vi "bac.vi"() -> ()   [LabVIEW 2019]
uses:
  <vilib>/Rock Robotics/WPI/ThirdParty/Phoenix-LabVIEW/Motor Controller/Controls/CTRE_Phoenix_MotorControl_ControlMode.ctl
  <vilib>/Rock Robotics/WPI/ThirdParty/Phoenix-LabVIEW/Motor Controller/Get/CTRE_Phoenix_MotorController_GetQuadratureData.vi
  <vilib>/Rock Robotics/Network Tables/NT Read Boolean.vi
  <vilib>/Rock Robotics/Network Tables/NT Read Number.vi
  Robot Global Data.vi
  <vilib>/Rock Robotics/Network Tables/NT Write Boolean.vi
  <vilib>/Rock Robotics/Network Tables/NT Write Number.vi
panel:
  out "Quadrature Position":i32
  out "Switch Pressed 3":bool
  out "Switch Pressed 2":bool
  out "Switch Pressed":bool
  in  "State":i8
  in  "Motor Speed":dbl=1.0
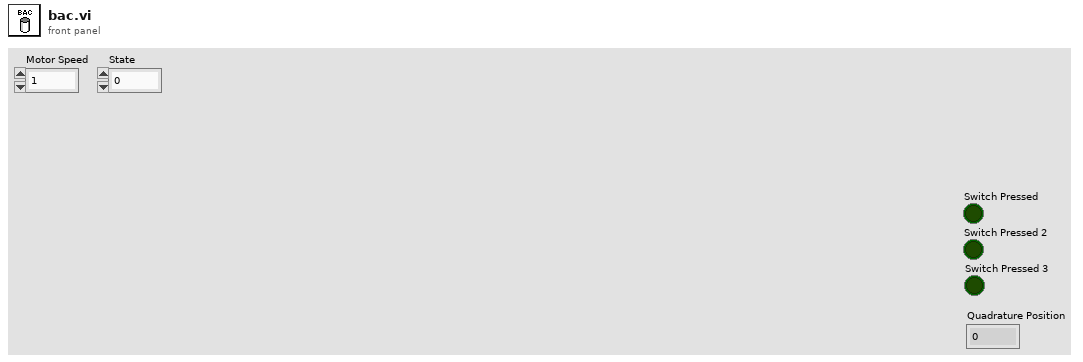
[diagram p1: front panel]
types:
  T1 = typedef "CTRE_Phoenix_MotorControl_ControlMode.ctl" = u16
  T2 = typedef "WPI_SwitchDevRef.ctl" = cluster{"DevStatus":errorcluster, "DIO Channel":T3, "CntIndex":T4, "Normally Closed":bool}
  T3 = typedef "FPGA_DIOChannel.ctl" = enum8{"DIO 0", "DIO 1", "DIO 2", "DIO 3", "DIO 4", "DIO 5", "DIO 6", "DIO 7", "DIO 8", "DIO 9", "DIO MXP 0", "DIO MXP 1", "DIO MXP 2", "DIO MXP 3", "DIO MXP 4", "DIO MXP 5", "DIO MXP 6", "DIO MXP 7", "DIO MXP 8", "DIO MXP 9", "DIO MXP 10", "DIO MXP 11", "DIO MXP 12", "DIO MXP 13", "DIO MXP 14", "DIO MXP 15", "SPI Port CS1", "SPI Port CS2", "SPI Port CS3", "SPI Port MISO", "SPI Port MOSI", "Invalid"}
  T4 = typedef "FPGA_CounterCtrSystemIndex.ctl" = enum8{"Ctr 0", "Ctr 1", "Ctr 2", "Ctr 3", "Ctr 4", "Ctr 5", "Ctr 6", "Ctr 7", "Invalid"}
  T5 = typedef "WPI_MotorControlDeviceRef.ctl" = cluster{"DeviceStatus":errorcluster, "Type":T6, "PWM":cluster{"PWM Channel":T7, "DeadBand":T8}, "CAN":cluster{"Device Number":u8, "SetOutput VI Ref":variant, "GetOutput VI Ref":variant, "Enable VI Ref":variant, "Disable VI Ref":variant, "Data":variant}, "Invert":bool, "DIO PWM":cluster{"PWM \"Enable\" Channel":T7, "DIOChannel":T3, "PWM Rate":dbl}}
  T6 = typedef "WPI_MotorControlType.ctl" = enum16{"PWM", "CAN", "DIO PWM"}
  T7 = typedef "FPGA_DIOPWMChannel.ctl" = enum8{"PWM 0", "PWM 1", "PWM 2", "PWM 3", "PWM 4", "PWM 5", "PWM 6", "PWM 7", "PWM 8", "PWM 9", "PWM MXP 0", "PWM MXP 1", "PWM MXP 2", "PWM MXP 3", "PWM MXP 4", "PWM MXP 5", "PWM MXP 6", "PWM MXP 7", "PWM MXP 8", "PWM MXP 9", "Invalid"}
  T8 = typedef "WPI_PWMDeadband.ctl" = cluster{"Name":string, "maxPositivePwm":i32, "minPositivePwm":i32, "centerPwm":i32, "maxNegativePwm":i32, "minNegativePwm":i32, "angularRange":u16}
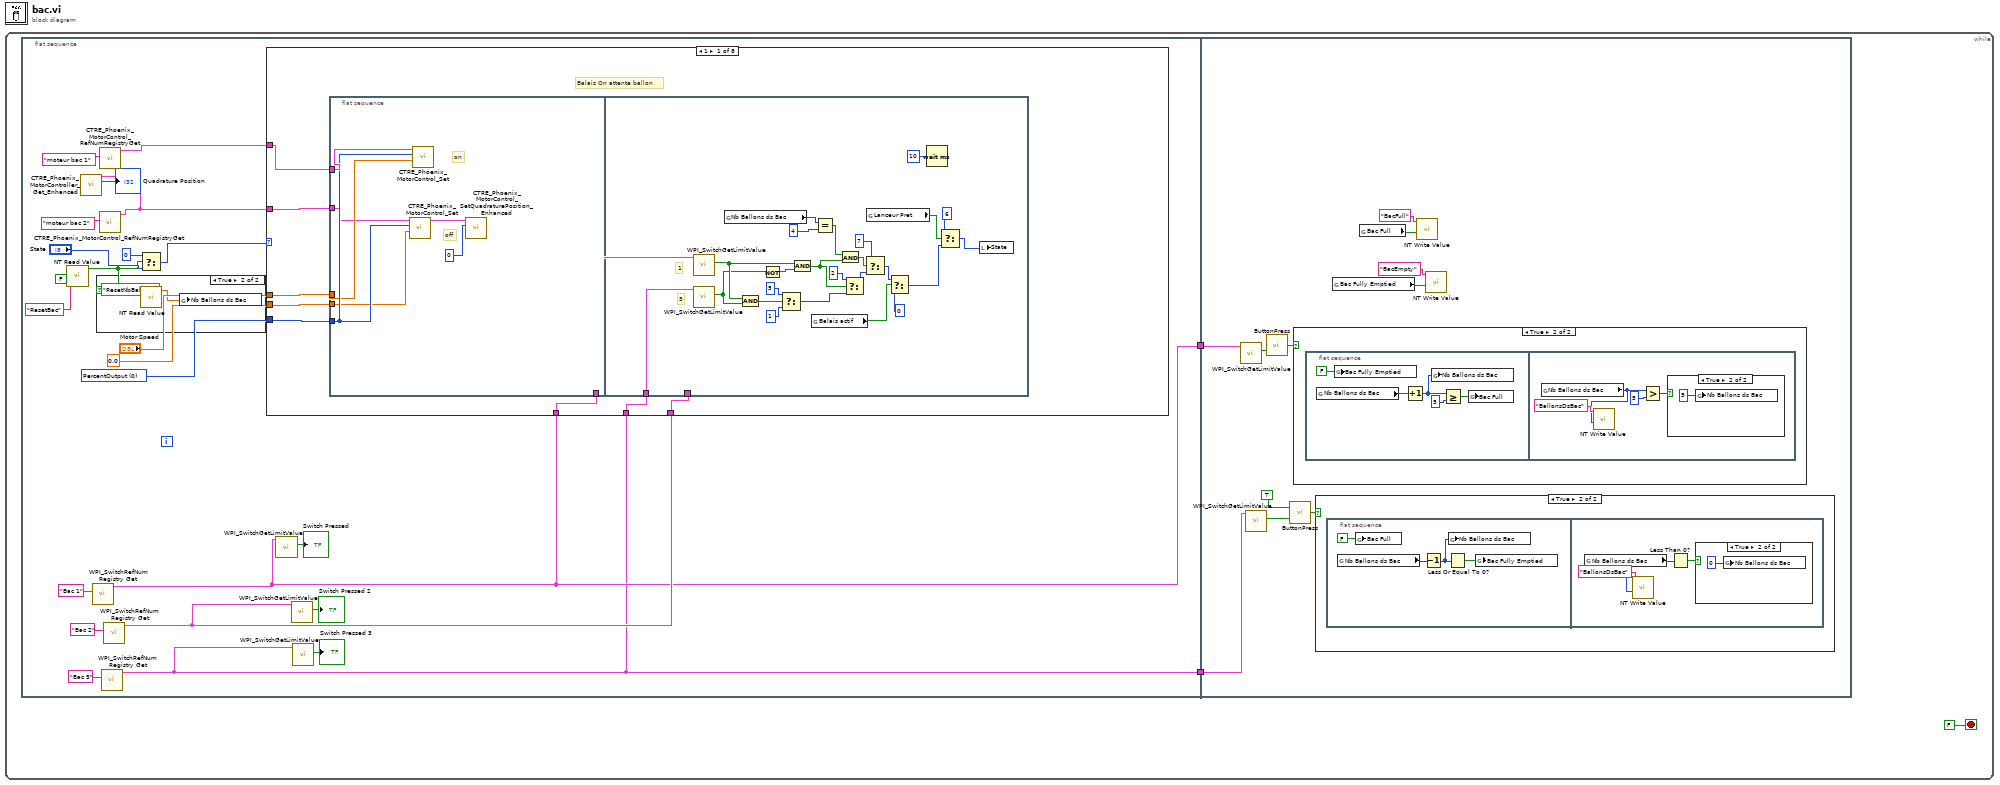
[diagram p0: block diagram]
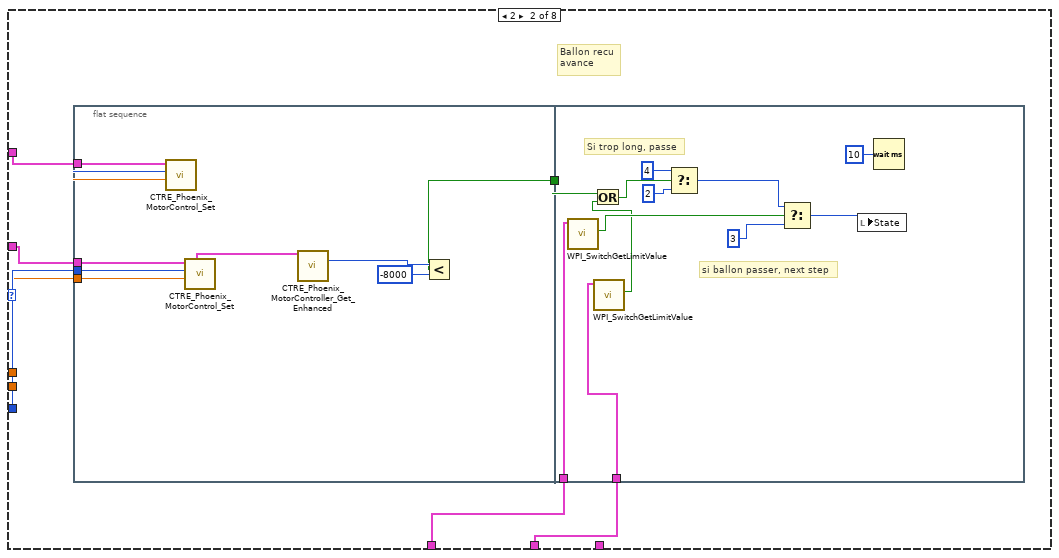
[diagram p3: hidden frame]
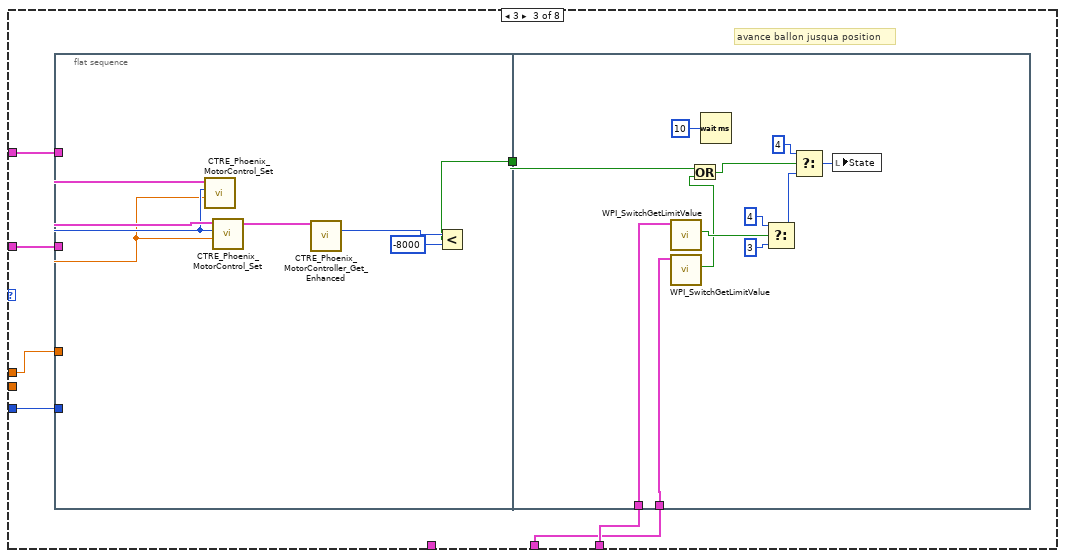
[diagram p4: hidden frame]
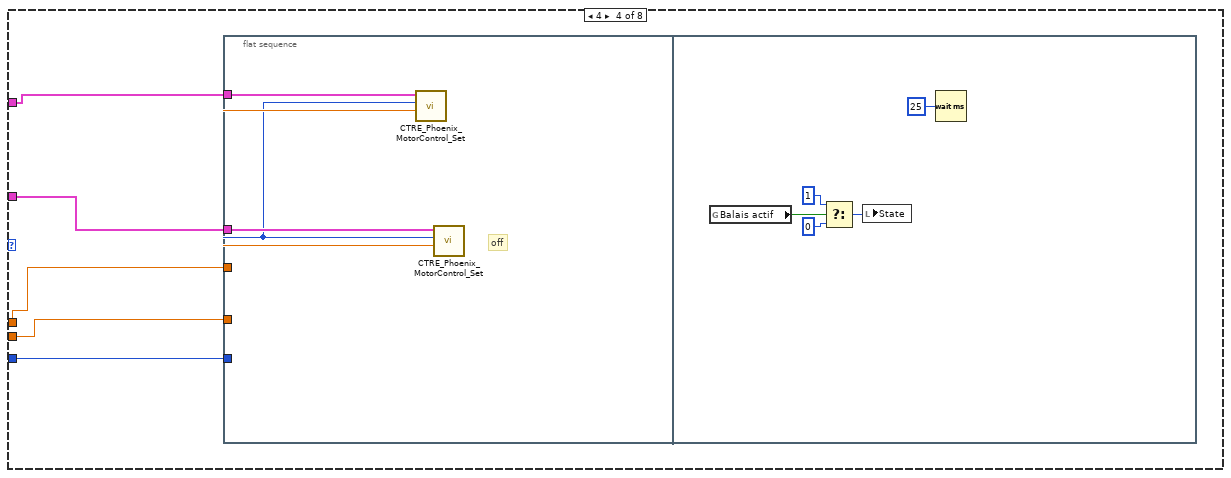
[diagram p5: hidden frame]
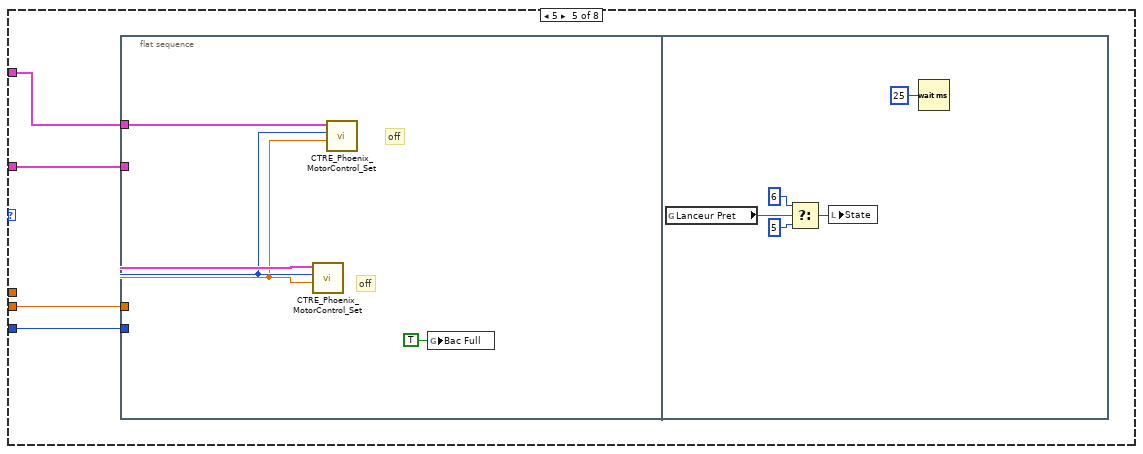
[diagram p6: hidden frame]
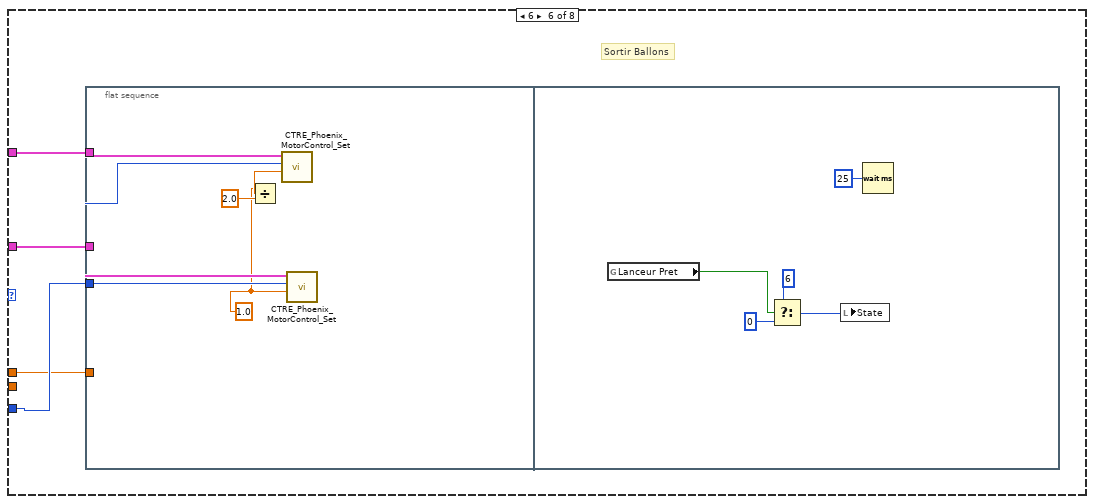
[diagram p7: hidden frame]
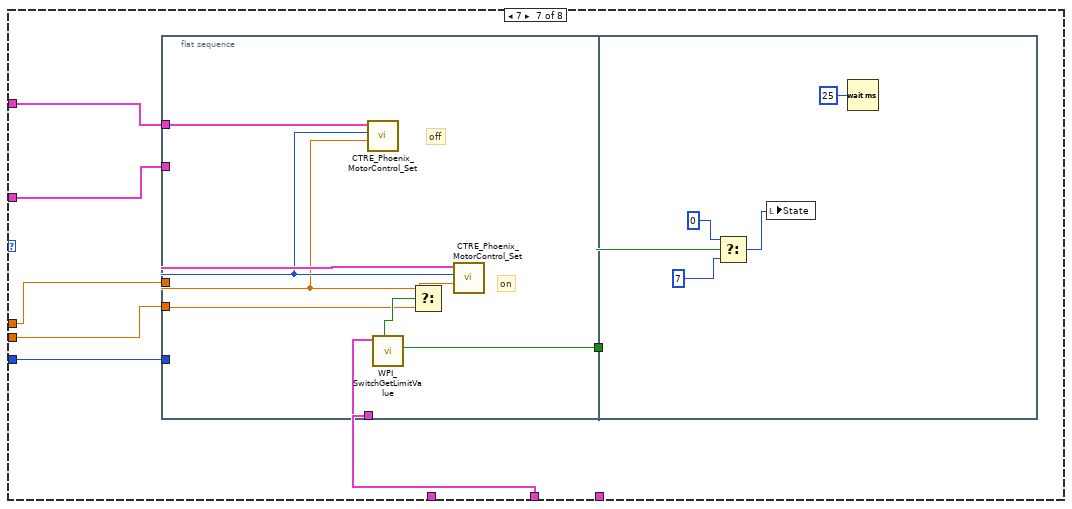
[diagram p8: hidden frame]
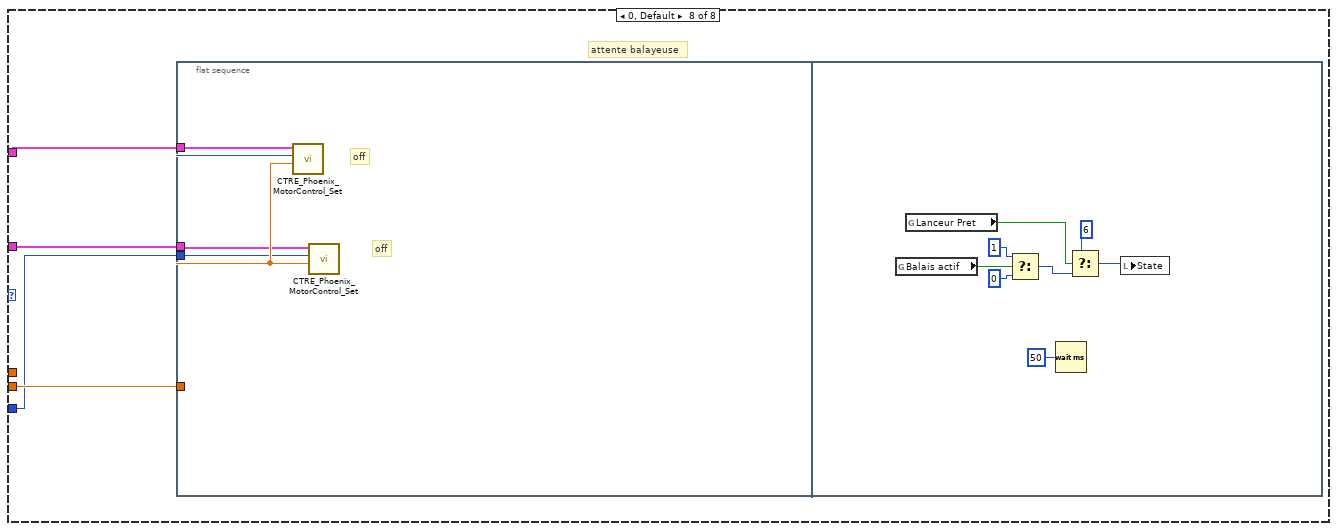
[diagram p9: hidden frame]
diagram:
  n1 = while {
    stop <- FALSE stop-if-true
    n2 = flat-sequence {
      tunnel: [w14] -> w2
      tunnel: [w11] -> w1
      tunnel: w2 -> [w208]
      tunnel: w1 -> [w207]
      frame #0 {
        w23 = T1 0 items=["PercentOutput"=0, "Position"=1, "Velocity"=2, "Current"=3, "Follower"=5, "MotionProfile"=6, "MotionMagic"=7, "MotionProfileArc"=10, "Disabled"=15] ("Control Mode")
        n3 = call-poly <vilib>:"NT Read Value.vi"("Default Value"=FALSE, "Name"="ResetBac") -> ("Boolean"=w4:bool)  [unwired: 8 in, 1 out]
        n4 = call <vilib>:"WPI_SwitchRefNum Registry Get.vi"("refnum name"="Bac 1") -> ("SwitchDevRef"=w14:T2)  [unwired: 9 in, 1 out]
        n5 = case shown="True" w4 {
          frame False {
          }
          frame True {
            n6 = call-poly <vilib>:"NT Read Value.vi"("Name"="ResetNbBallon") -> ("Numeric"=w27:dbl)  [unwired: 9 in, 1 out]
            n7 = global write "Robot Global Data.vi" "Nb Ballons ds Bac"(w27) -> ()
          }
        }
        n8 = call <vilib>:"CTRE_Phoenix_MotorControl_RefNumRegistryGet.vi"("refnum name"="moteur bac 2") -> ("PhoenixMotorControlDevRef"=w17:T5)  [unwired: 9 in, 1 out]
        n9 = call-poly <vilib>:"CTRE_Phoenix_MotorController_Get_Enhanced.vi"("PhoenixMotorControlDevRef"=w17) -> ("Quadrature Position"=→"Quadrature Position":i32)  [unwired: 11 in, 3 out]
        n10 = call <vilib>:"CTRE_Phoenix_MotorControl_RefNumRegistryGet.vi"("refnum name"="moteur bac 1") -> ("PhoenixMotorControlDevRef"=w25:T5)  [unwired: 9 in, 1 out]
        n11 = call <vilib>:"WPI_SwitchRefNum Registry Get.vi"("refnum name"="Bac 5") -> ("SwitchDevRef"=w11:T2)  [unwired: 9 in, 1 out]
        n12 = call <vilib>:"WPI_SwitchRefNum Registry Get.vi"("refnum name"="Bac 2") -> ("SwitchDevRef"=w16:T2)  [unwired: 9 in, 1 out]
        n13 = Select(t=i8 0, s=w4, f="State") -> (s? t:f=w5:i8)
        n14 = case shown="1" w5 {
          tunnel: w25 -> [w36 w75 w102 w126 w141 w155 w173 w190]
          tunnel: w23 -> [w35 w73 w100 w125 w139 w153 w169 w188]
          tunnel: 0.0 -> [w34 _ _ w124 w138 _ w171 w189]
          tunnel: "Motor Speed" -> [w33 w72 w99 w123 _ w152 w170 _]
          tunnel: w11 -> [w32 w69 w96 _ _ _ w168 _]
          tunnel: w17 -> [w30 w74 w101 w127 w140 w154 w172 w187]
          tunnel: w14 -> [w31 w71 _ _ _ _ _ _]
          tunnel: w16 -> [w29 _ w98 _ _ _ _ _]
          frame 1 {
            # "Balais On attente ballon"
            n15 = flat-sequence {
              tunnel: w36 -> [w43]
              tunnel: w35 -> [w42]
              tunnel: w34 -> [w41]
              tunnel: w33 -> [w40]
              tunnel: w30 -> [w39]
              tunnel: w32 -> [w64]
              tunnel: w31 -> [w63]
              tunnel: w29 -> [_]
              frame #0 {
                # "off"
                # "on"
                n16 = call <vilib>:"CTRE_Phoenix_MotorControl_Set.vi"("Output"=w41, "Control Mode"=w42, "PhoenixMotorControlDevRef"=w39) -> ("PhoenixMotorControlDevRef"=w38:T5)  [unwired: 7 in, 1 out]
                n17 = call <vilib>:"CTRE_Phoenix_MotorControl_Set.vi"("Output"=w40, "Control Mode"=w42, "PhoenixMotorControlDevRef"=w43) -> ()  [unwired: 7 in, 2 out]
                n18 = call <vilib>:"CTRE_Phoenix_MotorControl_SetQuadraturePosition_Enhanced.vi"("New Position"=0, "PhoenixMotorControlDevRef"=w38) -> ()  [unwired: 8 in, 2 out]
              }
              frame #1 {
                # "5"
                # "1"
                n19 = call <vilib>:"WPI_SwitchGetLimitValue.vi"("SwitchDevRef"=w63) -> ("Switch Pressed"=w62:bool)  [unwired: 8 in, 2 out]
                n20 = call <vilib>:"WPI_SwitchGetLimitValue.vi"("SwitchDevRef"=w64) -> ("Switch Pressed"=w61:bool)  [unwired: 8 in, 2 out]
                n21 = global read "Robot Global Data.vi" "Nb Ballons ds Bac"() -> (w51:u8)
                n22 = Compound Arithmetic op=AND(w62, w61) -> (w60:bool)
                n23 = Not(x=w61) -> (.not. x?=w65:bool)
                n24 = Select(t=i8 5, s=w60, f=i8 1) -> (s? t:f=w59:i8)
                n25 = And(x=w62, y=w65) -> (x .and. y?=w47:bool)
                n26 = global read "Robot Global Data.vi" "Balais actif"() -> (w54:bool)
                n27 = Equal?(x=w51, y=u8 4) -> (x = y?=w46:bool)
                n28 = And(x=w46, y=w47) -> (x .and. y?=w48:bool)
                n29 = Select(t=i8 2, s=w47, f=w59) -> (s? t:f=w49:i8)
                n30 = Select(t=i8 7, s=w48, f=w49) -> (s? t:f=w44:i8)
                n31 = global read "Robot Global Data.vi" "Lanceur Pret"() -> (w57:bool)
                n32 = Select(t=w44, s=w54, f=i8 0) -> (s? t:f=w53:i8)
                n33 = Wait (ms)(milliseconds to wait=u32 10) -> ()  [unwired: 1 out]
                n34 = Select(t=i8 6, s=w57, f=w53) -> (s? t:f=w55:i8)
                n35 = local write "State"(w55) -> ()
              }
            }
          }
          frame 2 {
            # "Ballon recu\navance"
            n36 = flat-sequence {
              tunnel: w75 -> [w83]
              tunnel: w74 -> [w82]
              tunnel: w73 -> [w81]
              tunnel: w72 -> [w80]
              tunnel: [w76] -> w70
              tunnel: w71 -> [w95]
              tunnel: w70 -> [w87]
              tunnel: w69 -> [w85]
              frame #0 {
                n37 = call <vilib>:"CTRE_Phoenix_MotorControl_Set.vi"("Output"=w80, "Control Mode"=w81, "PhoenixMotorControlDevRef"=w83) -> ()  [unwired: 7 in, 2 out]
                n38 = call <vilib>:"CTRE_Phoenix_MotorControl_Set.vi"("Output"=w80, "Control Mode"=w81, "PhoenixMotorControlDevRef"=w82) -> ("PhoenixMotorControlDevRef"=w77:T5)  [unwired: 7 in, 1 out]
                n39 = call-poly <vilib>:"CTRE_Phoenix_MotorController_Get_Enhanced.vi"("PhoenixMotorControlDevRef"=w77) -> ("Quadrature Position"=w79:i32)  [unwired: 11 in, 3 out]
                n40 = Less?(x=w79, y=-8000) -> (x < y?=w76:bool)
              }
              frame #1 {
                # "si ballon passer, next step"
                # "Si trop long, passe"
                n41 = call <vilib>:"WPI_SwitchGetLimitValue.vi"("SwitchDevRef"=w95) -> ("Switch Pressed"=w88:bool)  [unwired: 8 in, 2 out]
                n42 = call <vilib>:"WPI_SwitchGetLimitValue.vi"("SwitchDevRef"=w85) -> ("Switch Pressed"=w84:bool)  [unwired: 8 in, 2 out]
                n43 = Or(x=w87, y=w84) -> (x .or. y?=w86:bool)
                n44 = Select(t=i8 4, s=w86, f=i8 2) -> (s? t:f=w89:i8)
                n45 = Select(t=w89, s=w88, f=i8 3 ("t")) -> (s? t:f=w92:i8)
                n46 = local write "State"(w92) -> ()
                n47 = Wait (ms)(milliseconds to wait=u32 10) -> ()  [unwired: 1 out]
              }
            }
          }
          frame 3 {
            # "avance ballon jusqua position"
            n48 = flat-sequence {
              tunnel: w102 -> [w110]
              tunnel: w101 -> [w109]
              tunnel: w100 -> [w108]
              tunnel: w99 -> [w107]
              tunnel: [w103] -> w97
              tunnel: w98 -> [w122]
              tunnel: w97 -> [w113]
              tunnel: w96 -> [w115]
              frame #0 {
                n49 = call <vilib>:"CTRE_Phoenix_MotorControl_Set.vi"("Output"=w107, "Control Mode"=w108, "PhoenixMotorControlDevRef"=w110) -> ()  [unwired: 7 in, 2 out]
                n50 = call <vilib>:"CTRE_Phoenix_MotorControl_Set.vi"("Output"=w107, "Control Mode"=w108, "PhoenixMotorControlDevRef"=w109) -> ("PhoenixMotorControlDevRef"=w104:T5)  [unwired: 7 in, 1 out]
                n51 = call-poly <vilib>:"CTRE_Phoenix_MotorController_Get_Enhanced.vi"("PhoenixMotorControlDevRef"=w104) -> ("Quadrature Position"=w106:i32)  [unwired: 11 in, 3 out]
                n52 = Less?(x=w106, y=-8000) -> (x < y?=w103:bool)
              }
              frame #1 {
                n53 = call <vilib>:"WPI_SwitchGetLimitValue.vi"("SwitchDevRef"=w122) -> ("Switch Pressed"=w114:bool)  [unwired: 8 in, 2 out]
                n54 = call <vilib>:"WPI_SwitchGetLimitValue.vi"("SwitchDevRef"=w115) -> ("Switch Pressed"=w111:bool)  [unwired: 8 in, 2 out]
                n55 = Or(x=w113, y=w111) -> (x .or. y?=w112:bool)
                n56 = Wait (ms)(milliseconds to wait=u32 10) -> ()  [unwired: 1 out]
                n57 = Select(t=i8 4, s=w114, f=i8 3 ("t")) -> (s? t:f=w118:i8)
                n58 = Select(t=i8 4, s=w112, f=w118) -> (s? t:f=w117:i8)
                n59 = local write "State"(w117) -> ()
              }
            }
          }
          frame 4 {
            n60 = flat-sequence {
              tunnel: w127 -> [w132]
              tunnel: w126 -> [w131]
              tunnel: w125 -> [w128]
              tunnel: w124 -> [w130]
              tunnel: w123 -> [w129]
              frame #0 {
                # "off"
                n61 = call <vilib>:"CTRE_Phoenix_MotorControl_Set.vi"("Output"=w129, "Control Mode"=w128, "PhoenixMotorControlDevRef"=w131) -> ()  [unwired: 7 in, 2 out]
                n62 = call <vilib>:"CTRE_Phoenix_MotorControl_Set.vi"("Output"=w130, "Control Mode"=w128, "PhoenixMotorControlDevRef"=w132) -> ()  [unwired: 7 in, 2 out]
              }
              frame #1 {
                n63 = global read "Robot Global Data.vi" "Balais actif"() -> (w137:bool)
                n64 = Select(t=i8 1, s=w137, f=i8 0) -> (s? t:f=w134:i8)
                n65 = local write "State"(w134) -> ()
                n66 = Wait (ms)(milliseconds to wait=u32 25) -> ()  [unwired: 1 out]
              }
            }
          }
          frame 5 {
            n67 = flat-sequence {
              tunnel: w141 -> [w146]
              tunnel: w140 -> [w145]
              tunnel: w139 -> [w144]
              tunnel: w138 -> [w143]
              frame #0 {
                # "off"
                # "off"
                n68 = call <vilib>:"CTRE_Phoenix_MotorControl_Set.vi"("Output"=w143, "Control Mode"=w144, "PhoenixMotorControlDevRef"=w145) -> ()  [unwired: 7 in, 2 out]
                n69 = call <vilib>:"CTRE_Phoenix_MotorControl_Set.vi"("Output"=w143, "Control Mode"=w144, "PhoenixMotorControlDevRef"=w146) -> ()  [unwired: 7 in, 2 out]
                n70 = global write "Robot Global Data.vi" "Bac Full"(TRUE ("Bac Full")) -> ()
              }
              frame #1 {
                n71 = global read "Robot Global Data.vi" "Lanceur Pret"() -> (w147:bool)
                n72 = Select(t=i8 6, s=w147, f=i8 5) -> (s? t:f=w149:i8)
                n73 = local write "State"(w149) -> ()
                n74 = Wait (ms)(milliseconds to wait=u32 25) -> ()  [unwired: 1 out]
              }
            }
          }
          frame 6 {
            # "Sortir Ballons"
            n75 = flat-sequence {
              tunnel: w155 -> [w161]
              tunnel: w154 -> [w160]
              tunnel: w153 -> [w159]
              tunnel: w152 -> [_]
              frame #0 {
                w156 = 1.0 ("Output")
                n76 = Divide(x=w156, y=2.0) -> (x/y=w158:dbl)
                n77 = call <vilib>:"CTRE_Phoenix_MotorControl_Set.vi"("Output"=w158, "Control Mode"=w159, "PhoenixMotorControlDevRef"=w161) -> ()  [unwired: 7 in, 2 out]
                n78 = call <vilib>:"CTRE_Phoenix_MotorControl_Set.vi"("Output"=w156, "Control Mode"=w159, "PhoenixMotorControlDevRef"=w160) -> ()  [unwired: 7 in, 2 out]
              }
              frame #1 {
                n79 = global read "Robot Global Data.vi" "Lanceur Pret"() -> (w165:bool)
                n80 = Select(t=i8 6, s=w165, f=i8 0) -> (s? t:f=w162:i8)
                n81 = local write "State"(w162) -> ()
                n82 = Wait (ms)(milliseconds to wait=u32 25) -> ()  [unwired: 1 out]
              }
            }
          }
          frame 7 {
            n83 = flat-sequence {
              tunnel: w173 -> [w181]
              tunnel: w172 -> [w180]
              tunnel: w171 -> [w174]
              tunnel: w170 -> [w175]
              tunnel: w169 -> [w179]
              tunnel: w168 -> [w178]
              tunnel: [w176] -> w167
              tunnel: w167 -> [w182]
              frame #0 {
                # "on"
                # "off"
                n84 = call <vilib>:"CTRE_Phoenix_MotorControl_Set.vi"("Output"=w174, "Control Mode"=w179, "PhoenixMotorControlDevRef"=w181) -> ()  [unwired: 7 in, 2 out]
                n85 = call <vilib>:"WPI_SwitchGetLimitValue.vi"("SwitchDevRef"=w178) -> ("Switch Pressed"=w176:bool)  [unwired: 8 in, 2 out]
                n86 = Select(t=w174, s=w176, f=w175) -> (s? t:f=w177:dbl)
                n87 = call <vilib>:"CTRE_Phoenix_MotorControl_Set.vi"("Output"=w177, "Control Mode"=w179, "PhoenixMotorControlDevRef"=w180) -> ()  [unwired: 7 in, 2 out]
              }
              frame #1 {
                n88 = Select(t=i8 0, s=w182, f=i8 7 ("t")) -> (s? t:f=w184:i8)
                n89 = local write "State"(w184) -> ()
                n90 = Wait (ms)(milliseconds to wait=u32 25) -> ()  [unwired: 1 out]
              }
            }
          }
          frame 0, Default {
            # "attente balayeuse"
            n91 = flat-sequence {
              tunnel: w190 -> [w194]
              tunnel: w189 -> [w193]
              tunnel: w188 -> [w192]
              tunnel: w187 -> [w191]
              frame #0 {
                # "off"
                # "off"
                n92 = call <vilib>:"CTRE_Phoenix_MotorControl_Set.vi"("Output"=w193, "Control Mode"=w192, "PhoenixMotorControlDevRef"=w194) -> ()  [unwired: 7 in, 2 out]
                n93 = call <vilib>:"CTRE_Phoenix_MotorControl_Set.vi"("Output"=w193, "Control Mode"=w192, "PhoenixMotorControlDevRef"=w191) -> ()  [unwired: 7 in, 2 out]
              }
              frame #1 {
                n94 = global read "Robot Global Data.vi" "Balais actif"() -> (w202:bool)
                n95 = global read "Robot Global Data.vi" "Lanceur Pret"() -> (w198:bool)
                n96 = Select(t=i8 1, s=w202, f=i8 0) -> (s? t:f=w197:i8)
                n97 = Wait (ms)(milliseconds to wait=u32 50) -> ()  [unwired: 1 out]
                n98 = Select(t=i8 6, s=w198, f=w197) -> (s? t:f=w195:i8)
                n99 = local write "State"(w195) -> ()
              }
            }
          }
        }
        n100 = call <vilib>:"WPI_SwitchGetLimitValue.vi"("SwitchDevRef"=w14) -> ("Switch Pressed"=→"Switch Pressed":bool)  [unwired: 8 in, 2 out]
        n101 = call <vilib>:"WPI_SwitchGetLimitValue.vi"("SwitchDevRef"=w16) -> ("Switch Pressed"=→"Switch Pressed 2":bool)  [unwired: 8 in, 2 out]
        n102 = call <vilib>:"WPI_SwitchGetLimitValue.vi"("SwitchDevRef"=w11) -> ("Switch Pressed"=→"Switch Pressed 3":bool)  [unwired: 8 in, 2 out]
      }
      frame #1 {
        n103 = call <vilib>:"WPI_SwitchGetLimitValue.vi"("SwitchDevRef"=w208) -> ("Switch Pressed"=w210:bool)  [unwired: 8 in, 2 out]
        n104 = call <vilib>:"WPI_SwitchGetLimitValue.vi"("SwitchDevRef"=w207) -> ("Switch Pressed"=w212:bool)  [unwired: 8 in, 2 out]
        n105 = call "ButtonPress.vi"("Input"=w210) -> ("Output"=w211:bool)  [unwired: 1 in]
        n106 = call "ButtonPress.vi"("Input"=w212, "Falling Edge?"=TRUE) -> ("Output"=w213:bool)
        n107 = case shown="True" w211 {
          frame False {
          }
          frame True {
            n108 = flat-sequence {
              frame #0 {
                n109 = global read "Robot Global Data.vi" "Nb Ballons ds Bac"() -> (w224:u8)
                n110 = global write "Robot Global Data.vi" "Bac Fully Emptied"(FALSE ("Bac Fully Emptied")) -> ()
                n111 = Increment(x=w224) -> (x+1=w225:u8)
                n112 = global write "Robot Global Data.vi" "Nb Ballons ds Bac"(w225) -> ()
                n113 = Greater Or Equal?(x=w225, y=u8 5) -> (x >= y?=w226:bool)
                n114 = global write "Robot Global Data.vi" "Bac Full"(w226) -> ()
              }
              frame #1 {
                n115 = global read "Robot Global Data.vi" "Nb Ballons ds Bac"() -> (w227:u8)
                n116 = call-poly <vilib>:"NT Write Value.vi"("Numeric"=w227, "Name"="BallonsDsBac") -> ()  [unwired: 9 in, 1 out]
                n117 = Greater?(x=w227, y=u8 5) -> (0:w229:bool)
                n118 = case shown="True" w229 {
                  frame False {
                  }
                  frame True {
                    n119 = global write "Robot Global Data.vi" "Nb Ballons ds Bac"(u8 5 ("Nb Ballons ds Bac")) -> ()
                  }
                }
              }
            }
          }
        }
        n120 = case shown="True" w213 {
          frame False {
          }
          frame True {
            n121 = flat-sequence {
              frame #0 {
                n122 = global read "Robot Global Data.vi" "Nb Ballons ds Bac"() -> (w215:u8)
                n123 = global write "Robot Global Data.vi" "Bac Full"(FALSE ("Bac Full")) -> ()
                n124 = Decrement(x=w215) -> (x-1=w216:u8)
                n125 = Less Or Equal To 0?(x=w216) -> (x <= 0?=w217:bool)
                n126 = global write "Robot Global Data.vi" "Nb Ballons ds Bac"(w216) -> ()
                n127 = global write "Robot Global Data.vi" "Bac Fully Emptied"(w217) -> ()
              }
              frame #1 {
                n128 = global read "Robot Global Data.vi" "Nb Ballons ds Bac"() -> (w218:u8)
                n129 = call-poly <vilib>:"NT Write Value.vi"("Numeric"=w218, "Name"="BallonsDsBac") -> ()  [unwired: 9 in, 1 out]
                n130 = Less Than 0?(x=w218) -> (x < 0?=w220:bool)
                n131 = case shown="True" w220 {
                  frame False {
                  }
                  frame True {
                    n132 = global write "Robot Global Data.vi" "Nb Ballons ds Bac"(u8 0 ("Nb Ballons ds Bac")) -> ()
                  }
                }
              }
            }
          }
        }
        n133 = global read "Robot Global Data.vi" "Bac Fully Emptied"() -> (w205:bool)
        n134 = global read "Robot Global Data.vi" "Bac Full"() -> (w206:bool)
        n135 = call-poly <vilib>:"NT Write Value.vi"("Boolean"=w206, "Name"="BacFull") -> ()  [unwired: 9 in, 1 out]
        n136 = call-poly <vilib>:"NT Write Value.vi"("Boolean"=w205, "Name"="BacEmpty") -> ()  [unwired: 9 in, 1 out]
      }
    }
  }
